vi "WSVCAP SHL FPGA LL Procedure RFFE - Send SSC.vi"(0 "Procedure Step":T1, 1 "Wait Ticks Remaining":u32, 5 "Wait Ticks":u32, 11 "error in (no error)":errorcluster, 13 "Socket Mask":u32) -> (3 "Wait Ticks Remaining Out":u32, 4 "Procedure Step Out":T1, 10 "Finished":bool, 15 "error out":errorcluster)   [LabVIEW 2012]
uses:
  Type Defs/WSVCAP SHL Procedure Step Enum.ctl
  Type Defs/WSVCAP SHL RFFE Write Line Enum.ctl
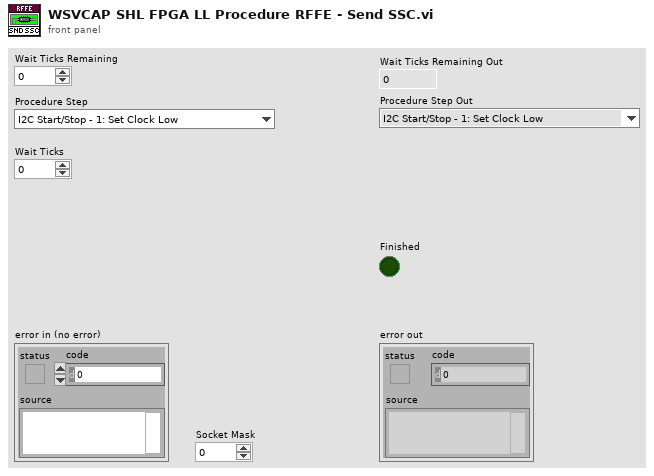
[diagram p1: front panel]
types:
  T1 = typedef "WSVCAP SHL Procedure Step Enum.ctl" = enum16{"I2C Start/Stop - 1: Set Clock Low", "I2C Start/Stop - 2: Wait", "I2C Start/Stop - 3: Set Data I", "I2C Start/Stop - 4: Wait", "I2C Start/Stop - 5: Set Clock High", "I2C Start/Stop - 6: Wait", "I2C Start/Stop - 7: Set Data II", "I2C Start/Stop - 8: Wait", "I2C Start/Stop - 9: Set Clock Low", "I2C Start/Stop - 10: Wait", "I2C Read ACK - 1: Set Clock High", "I2C Read ACK - 2: Wait", "I2C Read ACK - 3: Read ACK Bit", "I2C Read ACK - 4: Wait", "I2C Read ACK - 5: Set Clock Low", "I2C Read ACK - 6: Wait", "I2C Write ACK - 1: Write ACK Bit", "I2C Write ACK - 2: Wait", "I2C Write ACK - 3: Set Clock High", "I2C Write ACK - 4: Wait", "I2C Write ACK - 5: Set Clock Low", "I2C Write ACK - 6: Wait", "I2C Write ACK - 7: Set Data Low", "I2C Send Add - 1: Reset Bits Remaining", "I2C Send Add - 2: Set Data Bit", "I2C Send Add - 3: Wait", "I2C Send Add - 4: Set Clock High", "I2C Send Add - 5: Wait", "I2C Send Add - 6: Set Clock Low", "I2C Send Add - 7: Wait", "I2C Send Add - 8: Check Bits Remaining", "I2C Send Data - 1: Reset Bits Remaining", "I2C Send Data - 2: Load Write Bit from FIFO", "I2C Send Data - 3: Set Data Bit", "I2C Send Data - 4: Wait", "I2C Send Data - 5: Set Clock High", "I2C Send Data - 6: Wait", "I2C Send Data - 7: Set Clock Low", "I2C Send Data - 8: Wait", "I2C Send Data - 9: Check Bits Remaining", "I2C Receive Data - 1: Reset Bits Remaining", "I2C Receive Data - 2: Wait", "I2C Receive Data - 3: Set Clock High", "I2C Receive Data - 4: Wait", "I2C Receive Data - 5: Read Data Bit", "I2C Receive Data - 6: Wait", "I2C Receive Data - 7: Set Clock Low", "I2C Receive Data - 8: Wait", "I2C Receive Data - 9: Check Bits Remaining", "SPI Clear Lines - 1:Clear", "SPI Send/Receive - 1: Load SDA - Clock Low", "SPI Send/Receive - 2: Wait", "SPI Send/Receive - 3: Load DATO - Clock High", "SPI Send/Receive - 4: Wait", "SPI Wait CMD Delay - 1:Wait", "RFFE Send SSC - 1:Set Low", "RFFE Send SSC - 2:Wait", "RFFE Send SSC - 3:Set SDA High", "RFFE Send SSC - 4:Wait", "RFFE Send SSC - 5:Set SDA Low", "RFFE Send SSC - 6:Wait", "RFFE Send Data - 1:Set SCL High", "RFFE Send Data - 2:Wait", "RFFE Send Data - 3:Set SCL Low", "RFFE Send Data - 4:Wait", "RFFE Send Data - 5:Set SCL High (P)", "RFFE Send Data - 6:Wait", "RFFE Send Data - 7:Set SCL Low (P)", "RFFE Send Data - 8:Wait", "RFFE Send Data - 9:Set SCL High (BP)", "RFFE Send Data - 10:Wait", "RFFE Send Data - 11:Set SCL Low (BP)", "RFFE Send Data - 12:Wait", "RFFE Receive Data - 1:Set SCL High", "RFFE Receive Data - 2:Wait", "RFFE Receive Data - 3:Set SCL Low", "RFFE Receive Data - 4:Wait", "RFFE Receive Data - 5:Set SCL High (BP)", "RFFE Receive Data - 6:Wait", "RFFE Receive Data - 7:Set SCL Low (BP)", "RFFE Receive Data - 8:Wait", "RFFE Wait CMD Delay - 1:Wait", "RFFE Clear Lines - 1:Clear"}
  T2 = typedef "WSVCAP SHL RFFE Write Line Enum.ctl" = enum16{"SDAA", "SCLK"}
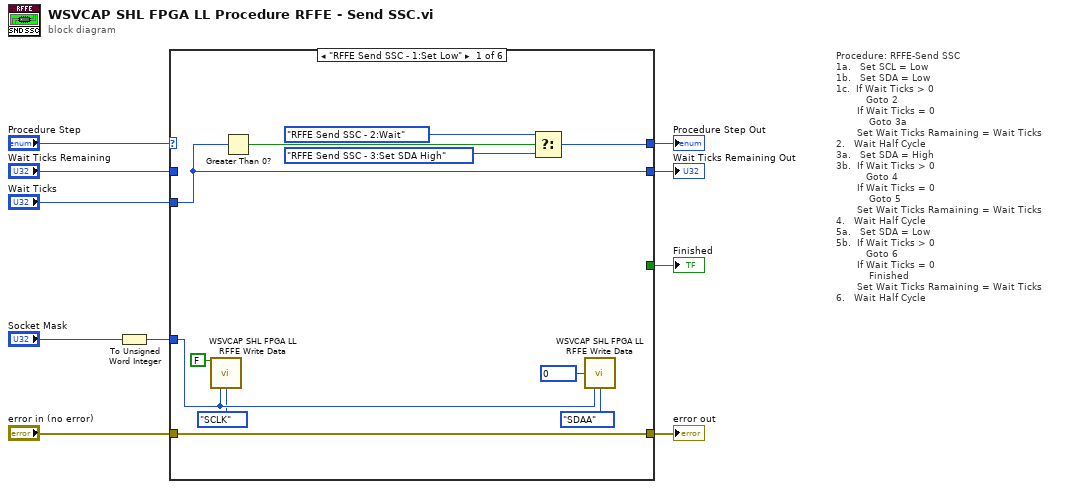
[diagram p0: block diagram]
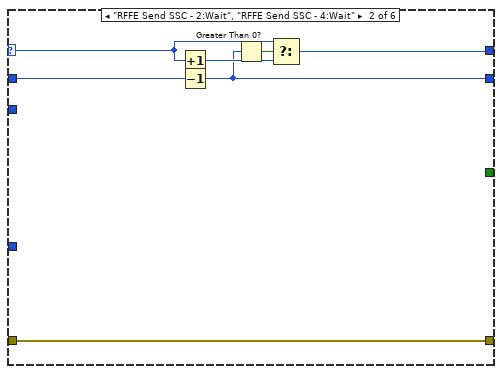
[diagram p2: hidden frame]
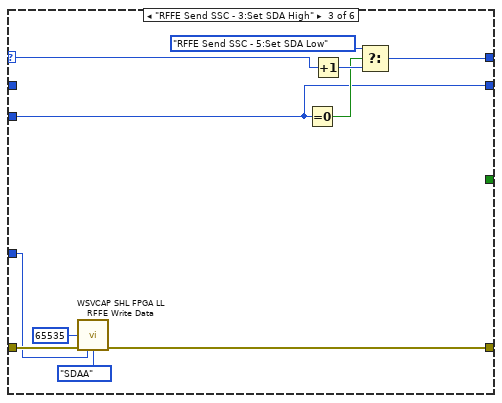
[diagram p3: hidden frame]
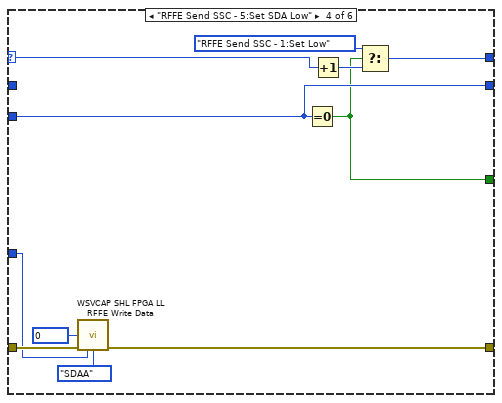
[diagram p4: hidden frame]
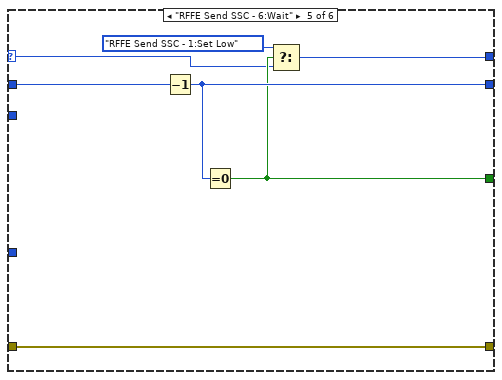
[diagram p5: hidden frame]
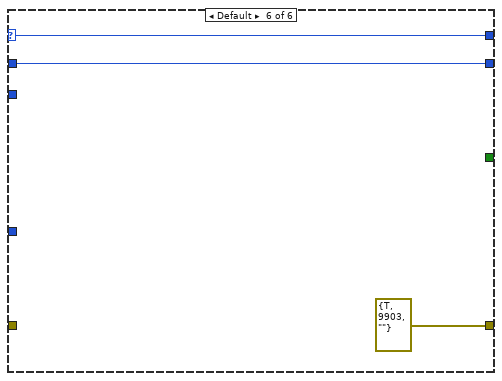
[diagram p6: hidden frame]
diagram:
  # "Procedure: RFFE-Send SSC\n1a.   Set SCL = Low\n1b.   Set SDA = Low\n1c.  If Wait Ticks > 0\n          Goto 2\n       If Wait Ticks = 0 \n           Goto 3a\n       Set Wait Ticks Ramaining = Wait Ticks\n2.   Wait Half Cycle\n3a.   Set SDA = High\n3b.  If Wait Ticks > 0\n          Goto 4\n       If Wait Ticks = 0 \n           Goto 5\n       Set Wait Ticks Ramaining = Wait Ticks\n4.   Wait Half Cycle\n5a.   Set SDA = Low\n5b.  If Wait Ticks > 0\n          Goto 6\n       If Wait Ticks = 0 \n           Finished\n       Set Wait Ticks Ramaining = Wait Ticks\n6.   Wait Half Cycle"
  n1 = To Unsigned Word Integer(number="Socket Mask") -> (unsigned 16bit integer=w7:u16)
  n2 = case shown="\"RFFE Send SSC - 1:Set Low\"" "Procedure Step" {
    selector: "Procedure Step" -> [_ w26 w39 w50 w51 w59]
    tunnel: [w19 w28 w36 w47 w57 errorcluster {"status"=TRUE, "code"=9903, "source"=""} ("error IO")] -> w9
    tunnel: "error in (no error)" -> [w19 w28 w37 w48 w57 _]
    tunnel: "Wait Ticks Remaining" -> [_ w24 _ _ w56 w58]
    tunnel: "Wait Ticks" -> [w15 _ w31 w43 _ _]
    tunnel: [_ _ _ w41 w53 _] -> w8
    tunnel: w7 -> [w14 _ w35 w46 _ _]
    tunnel: [w16 w23 w32 w44 w55 w59] -> w2
    tunnel: [w15 w22 w31 w43 w54 w58] -> w1
    frame "RFFE Send SSC - 1:Set Low" {
      n3 = call "WSVCAP SHL FPGA LL RFFE Write Data.vi"("CLK In"=FALSE ("Bit In"), "Socket Mask"=w14, "Line"=WSVCAP_SHL_RFFE_Write_Line_Enum."SCLK") -> ()  [unwired: 12 in, 1 out]
      n4 = Greater Than 0?(x=w15) -> (x > 0?=w20:bool)
      n5 = Select(t=WSVCAP_SHL_Procedure_Step_Enum."RFFE Send SSC - 2:Wait" ("Procedure Step"), s=w20, f=WSVCAP_SHL_Procedure_Step_Enum."RFFE Send SSC - 3:Set SDA High" ("Procedure Step")) -> (s? t:f=w16:T1)
      n6 = call "WSVCAP SHL FPGA LL RFFE Write Data.vi"("Data Word In"=u16 0, "Socket Mask"=w14, "Line"=WSVCAP_SHL_RFFE_Write_Line_Enum."SDAA") -> ()  [unwired: 12 in, 1 out]
    }
    frame "RFFE Send SSC - 2:Wait", "RFFE Send SSC - 4:Wait" {
      n7 = Increment(x=w26) -> (x+1=w25:T1)
      n8 = Decrement(x=w24) -> (x-1=w22:u32)
      n9 = Greater Than 0?(x=w22) -> (x > 0?=w27:bool)
      n10 = Select(t=w26, s=w27, f=w25) -> (s? t:f=w23:T1)
    }
    frame "RFFE Send SSC - 3:Set SDA High" {
      n11 = call "WSVCAP SHL FPGA LL RFFE Write Data.vi"("Data Word In"=u16 65535, "error in (no error)"=w37, "Socket Mask"=w35, "Line"=WSVCAP_SHL_RFFE_Write_Line_Enum."SDAA") -> ("error out"=w36:errorcluster)  [unwired: 11 in]
      n12 = Equal To 0?(x=w31) -> (x = 0?=w34:bool)
      n13 = Increment(x=w39) -> (x+1=w38:T1)
      n14 = Select(t=WSVCAP_SHL_Procedure_Step_Enum."RFFE Send SSC - 5:Set SDA Low" ("Procedure Step"), s=w34, f=w38) -> (s? t:f=w32:T1)
    }
    frame "RFFE Send SSC - 5:Set SDA Low" {
      n15 = call "WSVCAP SHL FPGA LL RFFE Write Data.vi"("Data Word In"=u16 0, "error in (no error)"=w48, "Socket Mask"=w46, "Line"=WSVCAP_SHL_RFFE_Write_Line_Enum."SDAA") -> ("error out"=w47:errorcluster)  [unwired: 11 in]
      n16 = Equal To 0?(x=w43) -> (x = 0?=w41:bool)
      n17 = Increment(x=w50) -> (x+1=w49:T1)
      n18 = Select(t=WSVCAP_SHL_Procedure_Step_Enum."RFFE Send SSC - 1:Set Low" ("Procedure Step"), s=w41, f=w49) -> (s? t:f=w44:T1)
    }
    frame "RFFE Send SSC - 6:Wait" {
      n19 = Decrement(x=w56) -> (x-1=w54:u32)
      n20 = Equal To 0?(x=w54) -> (x = 0?=w53:bool)
      n21 = Select(t=WSVCAP_SHL_Procedure_Step_Enum."RFFE Send SSC - 1:Set Low" ("f"), s=w53, f=w51) -> (s? t:f=w55:T1)
    }
    frame Default {
    }
  }
  "error out" <- w9
  "Finished" <- w8
  "Procedure Step Out" <- w2
  "Wait Ticks Remaining Out" <- w1
